vi "Configure DRAM Manager.vi"(0 "fpga interface in":refnum<k20>, 5 "serial channels":string[](array[string]), 7 "elements per dram bank":u32, 9 "dram arbiter config":T1={"write grant time (clocks)"=1000, "read grant time (clocks)"=1000}, 11 "error in (no error)":errorcluster, 12 "write time slice":u16=500, 13 "request time slice":u16=500) -> (4 "fpga interface out":refnum<k20>, 15 "error out":errorcluster)   [LabVIEW 2023, in "GettingStarted_Acq_148X_Host.lvlib"]
uses:
  GettingStarted_Acq_148X_Host.lvlib
  Types/148x_Acq_FPGA_Reference.ctl
  <vilib>/Utility/error.llb/Error Cluster From Error Code.vi
  <vilib>/rvi/errors/niLvFpgaAdjustHostInterfaceError.vi
  <vilib>/rvi/interface/nirviReadWriteControl/nirviReadWriteControl.xnode
  <vilib>/rvi/interface/Simulation/niFpgaSimulationCallBeginRW.vi
  NiFpgaLv.dll
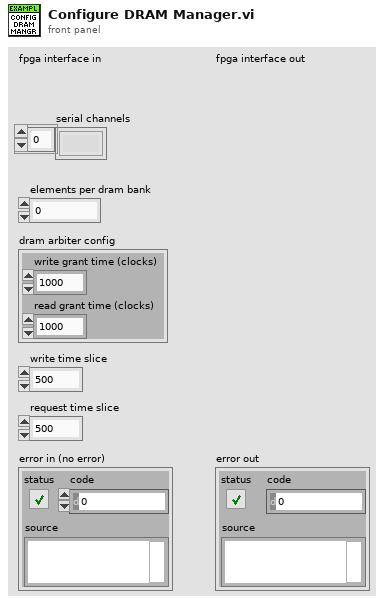
[diagram p1: front panel]
types:
  T1 = cluster{"write grant time (clocks)":u16, "read grant time (clocks)":u16}
  T2 = typedef "GettingStarted_Acq_148X_Host.lvlib/148x_Acq_FPGA_Reference.ctl" = refnum<k20>
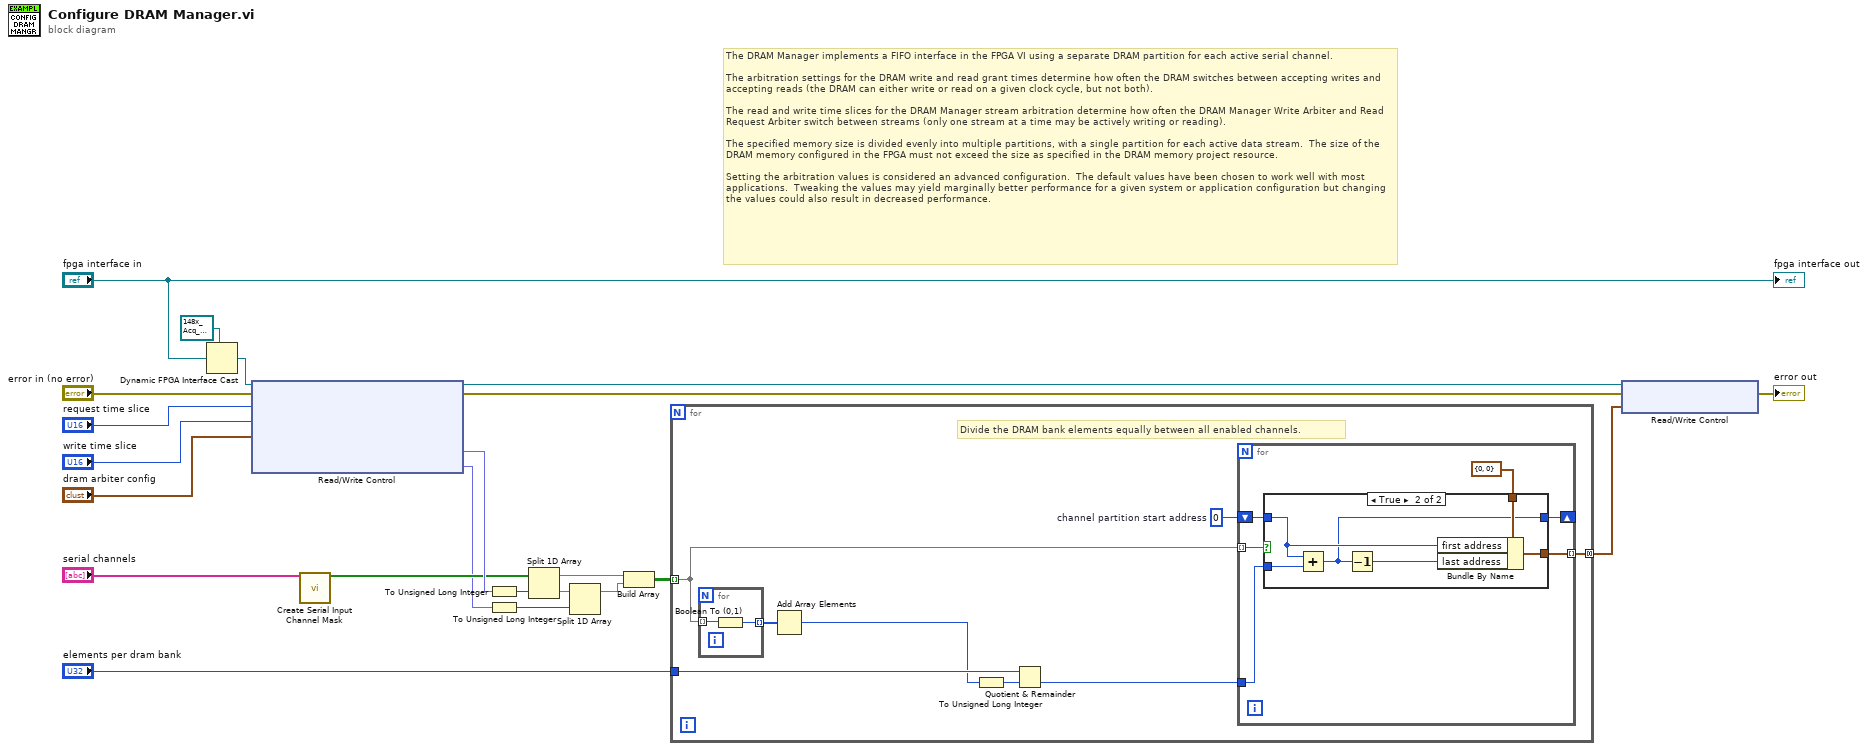
[diagram p0: block diagram]
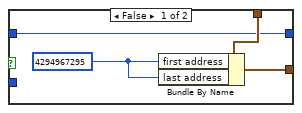
[diagram p2: hidden frame]
diagram:
  # "The DRAM Manager implements a FIFO interface in the FPGA VI using a separate DRAM partition for each active serial channel.  \n\nThe arbitration settings for the DRAM write and read grant times determine how often the DRAM switches between accepting writes and accepting reads (the DRAM can either write or read on a given clock cycle, but not both).  \n\nThe read and write time slices for the DRAM Manager stream arbitration determine how often the DRAM Manager Write Arbiter and Read Request Arbiter switch between streams (only one stream at a time may be actively writing or reading).  \n\nThe specified memory size is divided evenly into multiple partitions, with a single partition for each active data stream.  The size of the DRAM memory configured in the FPGA must not exceed the size as specified in the DRAM memory project resource.  \n\nSetting the arbitration values is considered an advanced configuration.  The default values have been chosen to work well with most applications.  Tweaking the values may yield marginally better performance for a given system or application configuration but changing the values could also result in decreased performance."
  n1 = Dynamic FPGA Interface Cast(Session In=T2 refnum ("FPGA VI Reference Out"), Type="fpga interface in") -> (Session Out=w10:T2)
  n2 = xnode "Read/Write Control"("FPGA VI Reference In"=w10, "error in"="error in (no error)", "request time slice"="request time slice", "write time slice"="write time slice", "dram arbiter config"="dram arbiter config") -> ("FPGA VI Reference Out"=w18:T2, "error out"=w16:errorcluster, "dram manager 0.num active streams"=w15:fxp<+,3,3>, "dram manager 1.num active streams"=w2:fxp<+,3,3>)
  n3 = call "Create Serial Input Channel Mask.vi"("serial channels"="serial channels") -> ("serial input channel mask"=w7:bool[])  [unwired: 14 in]
  n4 = To Unsigned Long Integer(number=w15) -> (unsigned 32bit integer=w4:u32)
  n5 = To Unsigned Long Integer(number=w2) -> (unsigned 32bit integer=w3:u32)
  n6 = Split 1D Array(array=w7, index=w4) -> (first subarray=w20:bool[], second subarray=w6:bool[])
  n7 = Split 1D Array(array=w6, index=w3) -> (first subarray=w5:bool[])  [unwired: 1 out]
  n8 = Build Array(w20, w5) -> (w19:bool[][])
  n9 = for {
    tunnel: "elements per dram bank" -> [w30]
    tunnel: w19 -> [w26] mode=indexing
    tunnel: [w23] -> w1 mode=concatenating
    w25 = u32 0  # channel partition start address
    # "Divide the DRAM bank elements equally between all enabled channels."
    n10 = for {
      tunnel: w26 -> [w48] mode=indexing
      tunnel: [w47] -> w28 mode=indexing
      n11 = Boolean To (0,1)(Boolean=w48) -> (0, 1=w47:i16)
    }
    n12 = Add Array Elements(numeric array=w28) -> (sum=w27:i16)
    n13 = To Unsigned Long Integer(number=w27) -> (unsigned 32bit integer=w29:u32)
    n14 = Quotient & Remainder(x=w30, y=w29) -> (floor(x/y)=w24:u32)  [unwired: 1 out]
    n15 = for {
      tunnel: w26 -> [w36] mode=indexing
      shift-right: [w33] -> _
      shift-left: w25 -> [w35]
      tunnel: w24 -> [w34]
      tunnel: [w32] -> w23 mode=indexing
      n16 = case shown="True" w36 {
        tunnel: [w39 w45] -> w32
        tunnel: cluster{"first address":u32, "last address":u32} {"first address"=0, "last address"=0} ("si 0 dram partition config") -> [w38 w46]
        tunnel: w35 -> [w37 w44]
        tunnel: w34 -> [_ w43]
        tunnel: [w37 w42] -> w33
        frame False {
          w40 = u32 4294967295 ("partition first address")
          n17 = Bundle By Name(cluster=w38, "first address"=w40, "last address"=w40) -> (w39:cluster{"first address":u32, "last address":u32})
        }
        frame True {
          n18 = Add(x=w44, y=w43) -> (x+y=w42:u32)
          n19 = Decrement(x=w42) -> (x-1=w41:u32)
          n20 = Bundle By Name(cluster=w46, "first address"=w44, "last address"=w41) -> (w45:cluster{"first address":u32, "last address":u32})
        }
      }
    }
  }
  n21 = xnode "Read/Write Control"("FPGA VI Reference In"=w18, "error in"=w16, "dram partition configs"=w1) -> ("error out"=→"error out":errorcluster)  [unwired: 1 out]
  "fpga interface out" <- "fpga interface in"
